vi "FTW-DevUtil-GenerateCloneName.vi"(0 "Fully qualified VI name":string="xyz.lvclass:abc.vi", 9 "Clone number (1)":i32=1) -> (4 "File name of clone VI":string, 6 "Clone VI numeric suffix":string, 10 "Fully qualified clone name":string)   [LabVIEW 2013]
doc: "Given the fully qualified name of a VI (meaning the name includes any library namespace prefixes), this VI returns the name of a clone of the VI. By default, it returns the name of the first clone that gets created, but you can request the Nth clone by supplying the \"Clone number\" input.\n\nUSE WITH CAUTION. The name returned by this VI can be used with the \"Open VI Reference\" function to open a VI reference to a clone VI. This is an unsupported feature of LabVIEW (i.e. opening an additional reference to a clone VI was never intended to work but someone forgot to disable it when clones were added to LabVIEW). Opening extra references beyond the one used to create the clone (i.e. the clone's \"this VI\" reference) is known to cause instabilities, including crashes, in some situations. However, such refnums are critical for writing certain debugging tools. Be careful.\n\nLabVIEW Task Manager v1.7.0.28\nRavi Beniwal (packaged by TimVargo) - LAVA\nCopyright (c) 2011-2014, Ravi Beniwal"
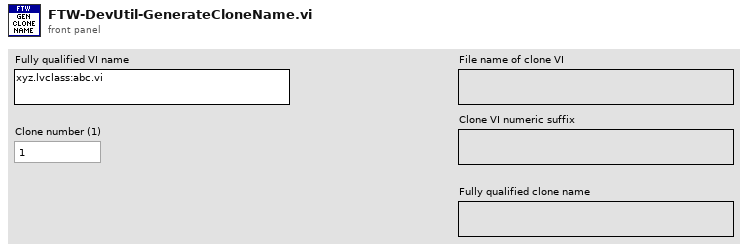
[diagram p1: front panel]
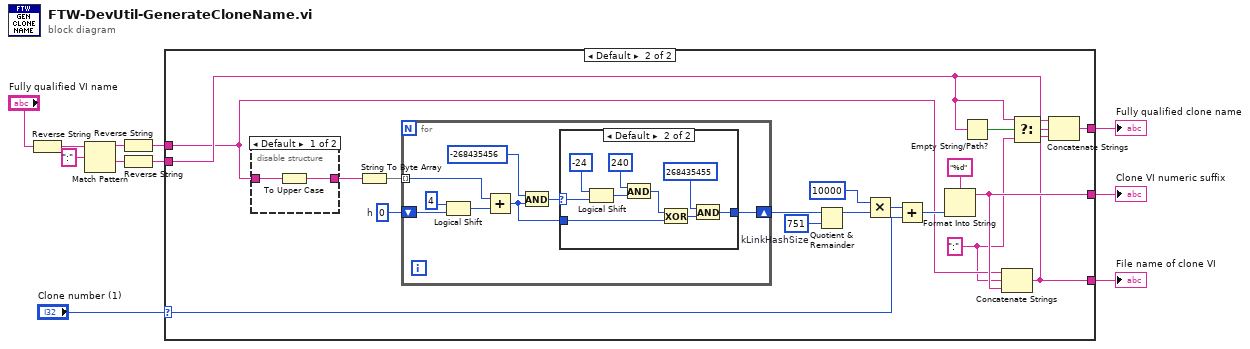
[diagram p0: block diagram]
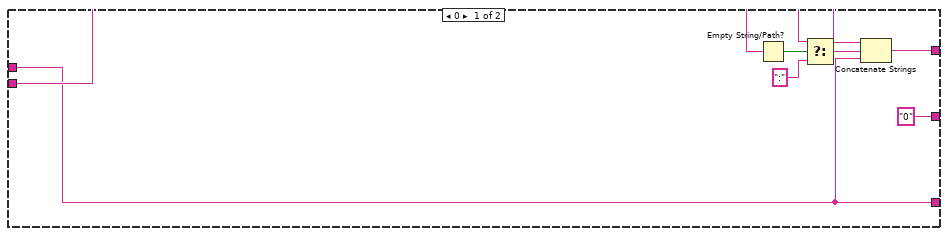
[diagram p2: hidden frame]
diagram:
  n1 = Reverse String(1:"Fully qualified VI name") -> (0:w4:string)
  n2 = Match Pattern(string=w4, regular expression=":") -> (before substring=w6:string, after substring=w7:string)  [unwired: 1 in, 2 out]
  n3 = Reverse String(1:w6) -> (0:w2:string)
  n4 = Reverse String(1:w7) -> (0:w1:string)
  n5 = case shown="Default" "Clone number (1)" {
    selector: "Clone number (1)" -> [_ w22]
    tunnel: [w12 w28] -> w11
    tunnel: ["0" w24] -> w10
    tunnel: [w13 w23] -> w9
    tunnel: w2 -> [w13 w20]
    tunnel: w1 -> [w14 w21]
    frame 0 {
      n6 = Empty String/Path?(string/path=w14) -> (empty?=w17:bool)
      n7 = Select(t=w14, s=w17, f=":") -> (s? t:f=w15:string)
      n8 = Concatenate Strings(w14, w15, w13) -> (w12:string)
    }
    frame Default {
      w19 = ":" ("string")
      w33 = 751  # kLinkHashSize
      w35 = 0  # h
      n9 = disable-structure shown="Default" {
        disable-tunnel: w20 -> [w57 _]
        disable-tunnel: [w56 _] -> w37
        frame condition #0 (active) {
          n10 = To Upper Case(1:w57) -> (0:w56:string)
        }
        frame condition #1 {
        }
      }
      n11 = String To Byte Array(string=w37) -> (unsigned byte array=w36:u8[])
      n12 = for {
        tunnel: w36 -> [w42] mode=indexing
        shift-right: [w38] -> w34
        shift-left: w35 -> [w45]
        n13 = Logical Shift(y=4, x=w45) -> (x << y=w43:i32)
        n14 = Add(x=w42, y=w43) -> (x+y=w39:i32)
        n15 = And(x=-268435456, y=w39) -> (x .and. y?=w40:i32)
        n16 = case shown="Default" w40 {
          selector: w40 -> [_ w55]
          tunnel: w39 -> [w46 w50]
          tunnel: [w46 w47] -> w38
          frame 0 {
          }
          frame Default {
            n17 = Logical Shift(y=-24, x=w55) -> (x << y=w53:i32)
            n18 = And(x=240, y=w53) -> (x .and. y?=w51:i32)
            n19 = Exclusive Or(1:w50, 2:w51) -> (0:w48:i32)
            n20 = And(x=268435455, y=w48) -> (x .and. y?=w47:i32)
          }
        }
      }
      n21 = Quotient & Remainder(x=w34, y=w33) -> (x-y*floor(x/y)=w32:i32)  [unwired: 1 out]
      n22 = Multiply(x=10000, y=w32) -> (x*y=w30:i32)
      n23 = Add(x=w30, y=w22) -> (x+y=w29:i32)
      n24 = Format Into String(format string="%d", w29) -> (resulting string=w24:string)  [unwired: 2 in, 1 out]
      n25 = Empty String/Path?(string/path=w21) -> (empty?=w26:bool)
      n26 = Concatenate Strings(w20, w19, w24) -> (w23:string)
      n27 = Select(t=w21, s=w26, f=w19) -> (s? t:f=w25:string)
      n28 = Concatenate Strings(w21, w25, w23) -> (w28:string)
    }
  }
  "File name of clone VI" <- w9
  "Fully qualified clone name" <- w11
  "Clone VI numeric suffix" <- w10
